vi "coerce.vi"(0 "GenericTrajectory in":refnum<class "TrajectoryDL091126GenericVoxel.lvclass">, 5 "x coordinates in":dbl[unit][](array[numeric]), 7 "y coordinates in":dbl[unit][](array[numeric]), 9 "z coordinates in":dbl[unit][](array[numeric]), 11 "error in (no error)":errorcluster) -> (4 "GenericTrajectory out":refnum<class "TrajectoryDL091126GenericVoxel.lvclass">, 6 "x coordinates out":dbl[unit][](array[numeric]), 8 "y coordinates out":dbl[unit][](array[numeric]), 10 "z coordinates out":dbl[unit][](array[numeric]), 14 "coerced?":bool[](array[boolean]), 15 "error out":errorcluster)   [LabVIEW 2010, in "TrajectoryDL091126GenericVoxel.lvclass"]
uses:
  TrajectoryDL091126GenericVoxel.lvclass
  common/enumerations/x_y_z_enumeration.ctl
  common/classes/ErrorController/ErrorController/class_data.vi
  common/classes/Box/Box/Box.lvclass
  common/classes/ErrorController/ErrorController/ErrorController.lvclass
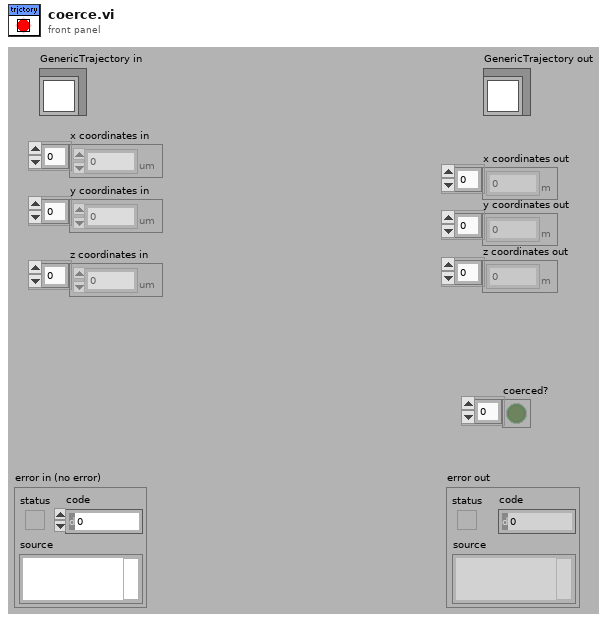
[diagram p1: front panel]
types:
  T1 = typedef "x_y_z_enumeration.ctl" = enum16{"x", "y", "z"}
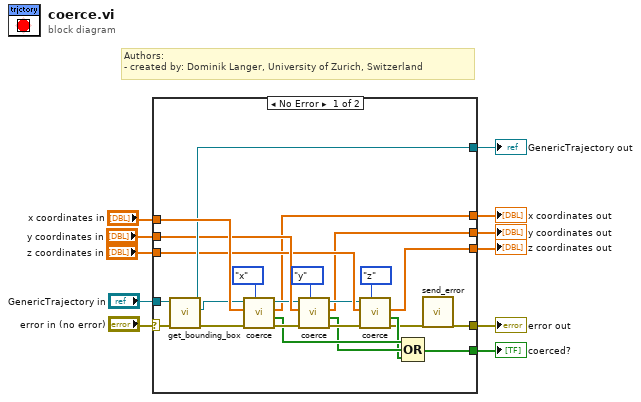
[diagram p0: block diagram]
diagram:
  # "Authors: \n- created by: Dominik Langer, University of Zurich, Switzerland"
  n1 = case shown="No Error" "error in (no error)" {
    selector: "error in (no error)" -> [w34 w37]
    tunnel: [w12 w37] -> w10
    tunnel: [w31 w36] -> w8
    tunnel: "GenericTrajectory in" -> [w32 w36]
    tunnel: "x coordinates in" -> [w35 _]
    tunnel: "y coordinates in" -> [w29 _]
    tunnel: "z coordinates in" -> [w28 _]
    tunnel: [w20 _] -> w4
    tunnel: [w19 _] -> w3
    tunnel: [w18 _] -> w2
    tunnel: [w15 _] -> w1
    frame No Error {
      n2 = call-dynamic "get_bounding_box.vi"("error in (no error)"=w34, "GenericTrajectory in"=w32) -> ("error out"=w33:errorcluster, "Box.lvclass"=w30:refnum<class "Box.lvclass">, "GenericTrajectory out"=w31:refnum<class "TrajectoryDL091126GenericVoxel.lvclass">)  [unwired: 7 in]
      n3 = call "coerce.vi"("dimension"=x_y_z_enumeration."x", "error in (no error)"=w33, "coordinates in"=w35, "Box in"=w30) -> ("error out"=w27:errorcluster, "coerced?"=w17:bool[], "coordinates out"=w20:dbl[unit][], "Box out"=w25:refnum<class "Box.lvclass">)  [unwired: 1 in, 3 out]
      n4 = call "coerce.vi"("dimension"=x_y_z_enumeration."y", "error in (no error)"=w27, "coordinates in"=w29, "Box in"=w25) -> ("error out"=w26:errorcluster, "coerced?"=w16:bool[], "coordinates out"=w19:dbl[unit][], "Box out"=w24:refnum<class "Box.lvclass">)  [unwired: 1 in, 3 out]
      n5 = call "coerce.vi"("dimension"=x_y_z_enumeration."z", "error in (no error)"=w26, "coordinates in"=w28, "Box in"=w24) -> ("error out"=w13:errorcluster, "coerced?"=w14:bool[], "coordinates out"=w18:dbl[unit][])  [unwired: 1 in, 4 out]
      n6 = Compound Arithmetic op=OR(w17, w16, w14) -> (w15:bool[])
      n7 = call "send_error.vi"("error in (no error)"=w13) -> ("error out"=w12:errorcluster)  [unwired: 10 in]
    }
    frame Error {
    }
  }
  "error out" <- w10
  "GenericTrajectory out" <- w8
  "coerced?" <- w1
  "x coordinates out" <- w4
  "y coordinates out" <- w3
  "z coordinates out" <- w2
